vi "CheckWorkload(SubVI).vi"(8 "error in (no error)":errorcluster, 11 "DVR Weekly/Country Data In":refnum<data-value>) -> (0 "error out":errorcluster, 2 "SRs Data Out":T1[](array[typedef]), 3 "DVR Weekly/Country Data Out":refnum<data-value>)   [LabVIEW 2017, in "DS_Lib.lvlib" / "SRReportParser.lvlib"]
uses:
  SRReportParser.lvlib
  TypeDefs/WeeklyData.ctl
  Modules/Private Controls/Data Raw.ctl
  TypeDefs/InWorkSR_Data.ctl
  Modules/Data Operations.lvlib
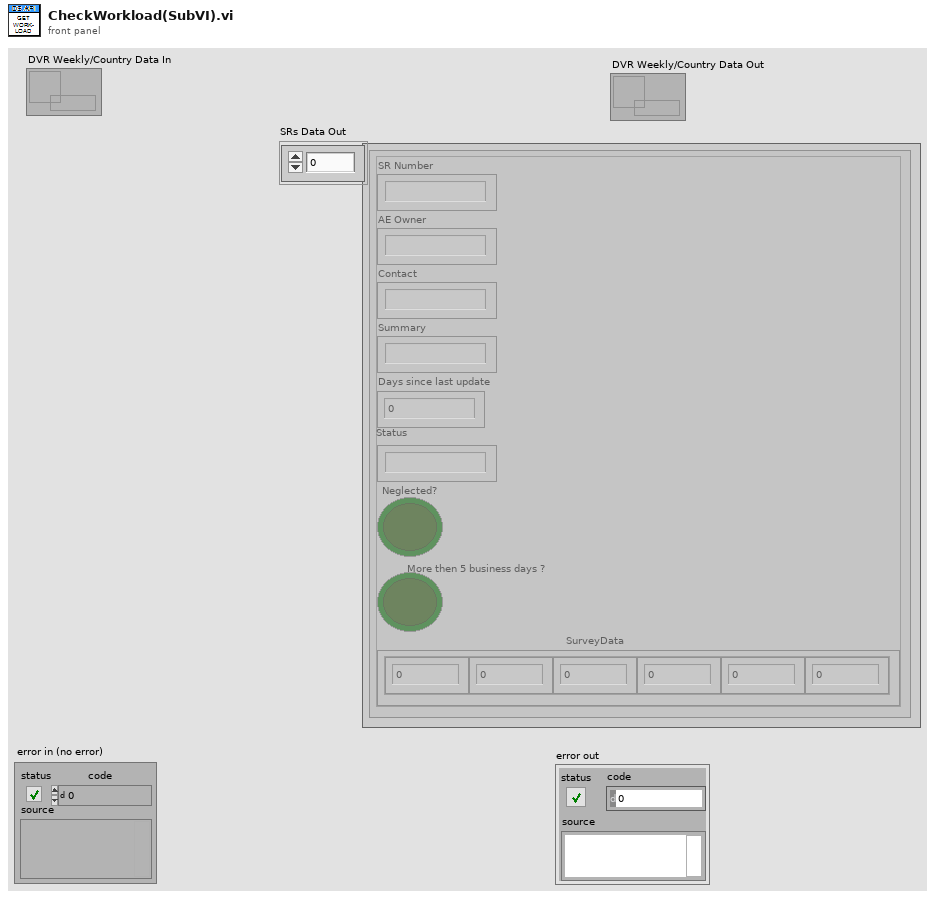
[diagram p1: front panel]
types:
  T1 = typedef "DS_Lib.lvlib/SRReportParser.lvlib/InWorkSR_Data.ctl" = cluster{"SR Number":string, "AE Owner":string, "Contact":string, "Summary":string, "Days since last update":dbl, "Status":string, "Neglected?":bool, "More then 5 business days ?":bool, "SurveyData":cluster{"Resolution Time":dbl, "Total Satisfaction":dbl, "Response Time":dbl, "Courtesy":dbl, "Problem Solved":dbl, "Level of effort":dbl}}
  T2 = typedef "DS_Lib.lvlib/SRReportParser.lvlib/WeeklyData.ctl" = cluster{"Week":u8, "AE-Romania":T3[], "AE-Poland":T3[], "AE-Hungary":T3[], "AE-Czech and Slovakia":T3[]}
  T3 = typedef "Data Operations.lvlib/Data Raw.ctl" = cluster{"SR Number":string, "Status":string, "Summary":string, "AE Owner":string, "AE Group":string, "Contact":string, "SurveyData":cluster{"Resolution Time":dbl, "Total Satisfaction":dbl, "Response Time":dbl, "Courtesy":dbl, "Problem Solved":dbl, "Level of effort":dbl}, "Time Data":cluster{"Last Update Date":timestamp, "Creation Date":timestamp, "Creation week":u8, "Last Update Week":u8}}
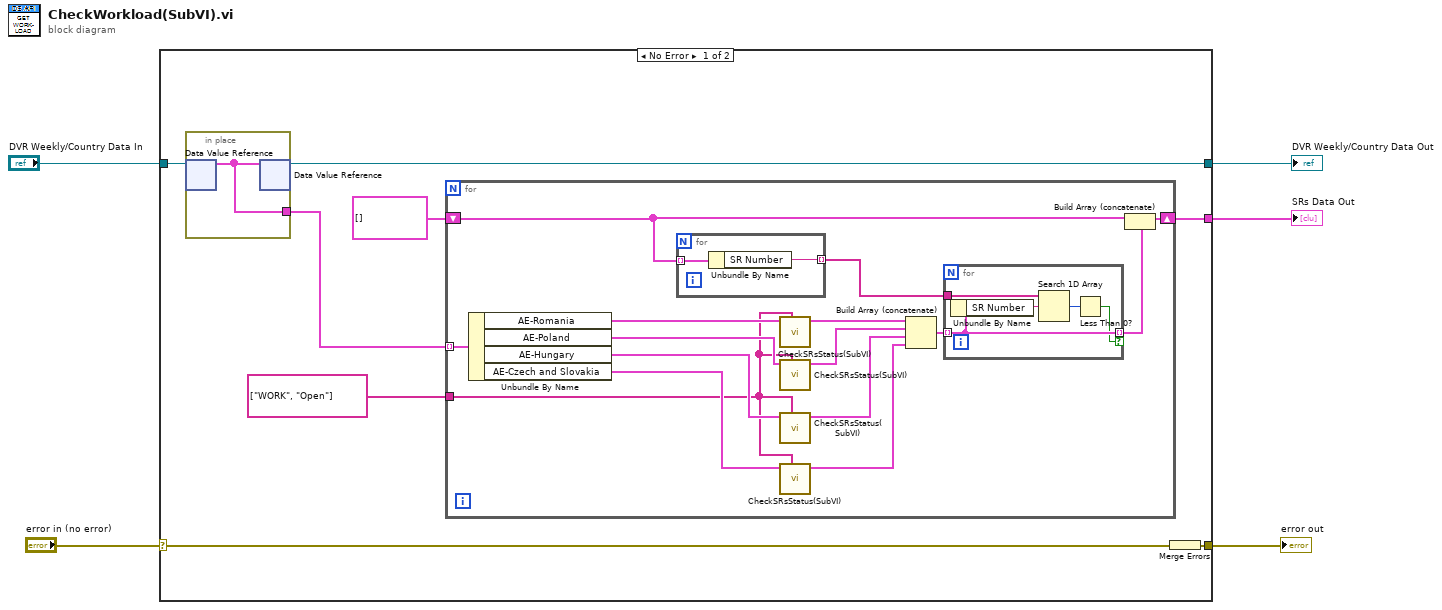
[diagram p0: block diagram]
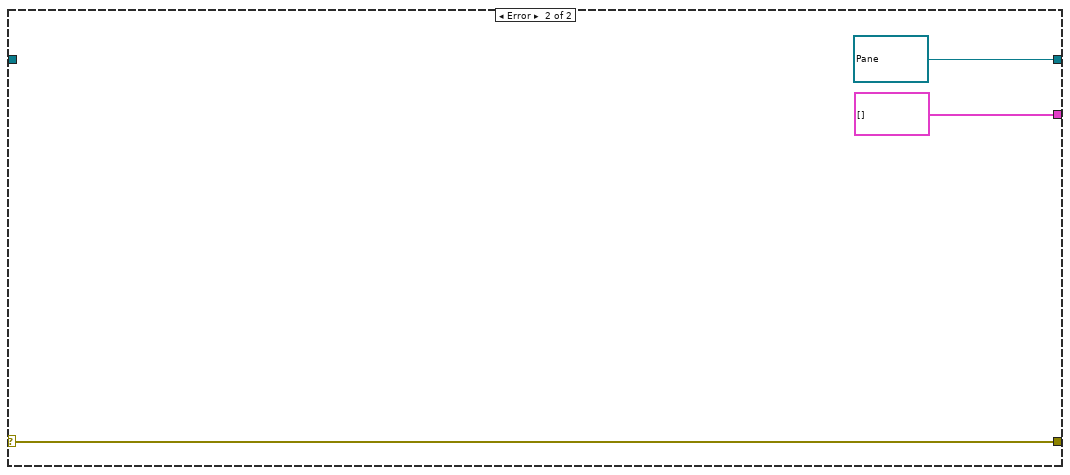
[diagram p2: hidden frame]
diagram:
  n1 = case shown="No Error" "error in (no error)" {
    selector: "error in (no error)" -> [w8 w39]
    tunnel: [w11 w39] -> w5
    tunnel: [w13 refnum<data-value> refnum ("data value reference")] -> w3
    tunnel: "DVR Weekly/Country Data In" -> [w12 _]
    tunnel: [w7 T1[] []] -> w1
    frame No Error {
      n2 = in-place {
        in-place-border: [w36] -> w10
        n3 = in-place-dvr #1(w12) -> (w36:T2[])  [unwired: 1 out]
        n4 = in-place-dvr #1(w36) -> (w13:refnum<data-value>)  [unwired: 1 out]
      }
      n5 = for {
        tunnel: w10 -> [w28] mode=indexing
        shift-right: [w15] -> w7
        shift-left: T1[] [] -> [w18]
        tunnel: string[] ["WORK", "Open"] ("Statuses") -> [w14]
        n6 = Unbundle By Name(w28) -> ("AE-Romania"=w27:T3[], "AE-Poland"=w26:T3[], "AE-Hungary"=w25:T3[], "AE-Czech and Slovakia"=w24:T3[])
        n7 = for {
          tunnel: w18 -> [w30] mode=indexing
          tunnel: [w29] -> w17 mode=indexing
          n8 = Unbundle By Name(w30) -> ("SR Number"=w29:string)
        }
        n9 = call "CheckSRsStatus(SubVI).vi"("Statuses"=w14, "AE-Group"=w27) -> ("SR Data Out"=w23:T1[])  [unwired: 8 in, 1 out]
        n10 = call "CheckSRsStatus(SubVI).vi"("Statuses"=w14, "AE-Group"=w26) -> ("SR Data Out"=w22:T1[])  [unwired: 8 in, 1 out]
        n11 = call "CheckSRsStatus(SubVI).vi"("Statuses"=w14, "AE-Group"=w25) -> ("SR Data Out"=w21:T1[])  [unwired: 8 in, 1 out]
        n12 = call "CheckSRsStatus(SubVI).vi"("Statuses"=w14, "AE-Group"=w24) -> ("SR Data Out"=w20:T1[])  [unwired: 8 in, 1 out]
        n13 = Build Array (concatenate)(w23, w22, w21, w20) -> (w19:T1[])
        n14 = for {
          tunnel: w19 -> [w33] mode=indexing
          tunnel: w17 -> [w35]
          tunnel: [w33] -> w16 mode=indexing if=w31
          n15 = Unbundle By Name(w33) -> ("SR Number"=w34:string)
          n16 = Search 1D Array(1D array=w35, element=w34) -> (index of element=w32:i32)  [unwired: 1 in]
          n17 = Less Than 0?(x=w32) -> (x < 0?=w31:bool)
        }
        n18 = Build Array (concatenate)(w18, w16) -> (w15:T1[])
      }
      n19 = Merge Errors(w8) -> (w11:errorcluster)
    }
    frame Error {
    }
  }
  "error out" <- w5
  "DVR Weekly/Country Data Out" <- w3
  "SRs Data Out" <- w1
